vi "Initialize.vi"(8 "error in":errorcluster, 11 "Plugin in":refnum<class "Digital Output Handler.lvclass">) -> (0 "error out":errorcluster, 3 "Plugin out":refnum<class "Digital Output Handler.lvclass">)   [LabVIEW 2023, in "Digital Output Handler.lvlib" / "Digital Output Handler.lvclass"]
uses:
  Digital Output Handler.lvclass
  C:/Program Files/National Instruments/LabVIEW 2023/vi.lib/FlexLogger/SDK/PluginSDK.lvlibp/PEFClasses/SDK/Plugin/Plugin.lvclass
  Digital Output Global.vi
  <vilib>/FlexLogger/SDK/PluginSDK.lvlibp/PEFClasses/SDK/Plugin/ParameterAccess/Write I32.vi
  <vilib>/FlexLogger/SDK/PluginSDK.lvlibp/PEFClasses/SDK/Plugin/Plugin.lvclass
  C:/Program Files/National Instruments/LabVIEW 2023/vi.lib/FlexLogger/SDK/PluginSDK.lvlibp/PEFClasses/SDK/Processing Element/Processing Element.lvclass
  C:/dev/niflexlogger-plugins/plugins/Digital Output Handler/source/Digital Output Handler/Digital Output Handler.lvclass
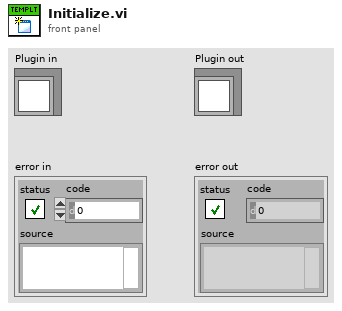
[diagram p1: front panel]
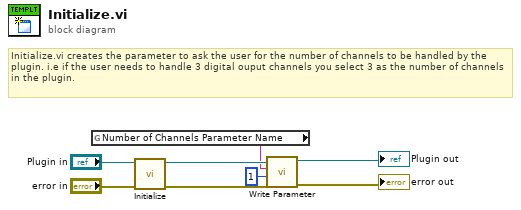
[diagram p0: block diagram]
diagram:
  # "Initialize.vi creates the parameter to ask the user for the number of channels to be handled by the plugin. i.e if the user needs to handle 3 digital ouput channels you select 3 as the number of channels in the plugin."
  n1 = global read "Digital Output Global.vi" "Number of Channels Parameter Name"() -> (w1:string)
  n2 = call-parent "Initialize.vi"("error in (no error)"="error in", "Plugin in"="Plugin in") -> ("error out"=w5:errorcluster, "Plugin out"=w4:refnum<class "Digital Output Handler.lvclass">)  [unwired: 8 in]
  n3 = call-poly <vilib>:"Write Parameter.vi"("error in (no error)"=w5, "Value"=1, "Name"=w1, "Plugin in"=w4) -> ("error out"=→"error out":errorcluster, "Plugin out"=→"Plugin out":refnum<class "Digital Output Handler.lvclass">)  [unwired: 6 in]
